vi "Binary to KLB(64-bit).vi"() -> ()   [LabVIEW 2013]
uses:
  File IO/KLB/VIs/Type Defs/KLB Settings Cluster.ctl
  File IO/KLB/VIs/Type Defs/KLB # of CPUs enum.ctl
  File IO/KLB/VIs/Type Defs/KLB compression type enum.ctl
  <vilib>/vision/Image Controls.llb/IMAQ Image.ctl
  File IO/KLB/KLB.lvlib
panel:
  in  "KLB Settings":T1={"Logical Cores"=enum."8", "pixelSize (um)"=[1.0, 1.0, 1.0, 1.0, 1.0], "blockSize"=[200, 197, 1, 1, 1], "compressionType"=enum."BZip2", "metadata"=""} {"pixelSize (um)" min=0.01 max=10 step=0.01 format="%.2f"}
  in  "Images per Chunk":u32=1
  out "Image":T4(plugin-control)
  out "KLB Conversion Time (ms)":u32=53091
  out "Image/Sector Size(bytes)":i64=3384359664
  in  "stop":bool
  out "Progress":u64(slide)=3579 max=5098 scale=0.0..3579.0
  out "Partial images in file?":bool
  out "# of Images":u32=3579
  out "error IO":errorcluster
  out "Height":u32=788
  out "Width":u32=1200
  in  "Created Image Path":path=path "G:/StreamingVideo/20150427_testStreamingVideoToDisk/09-25-2015_16-04-04-04 conv.klb"
  in  "Binary File":path=path "G:/StreamingVideo/20150427_testStreamingVideoToDisk/09-25-2015_16-04-04-04.bin"
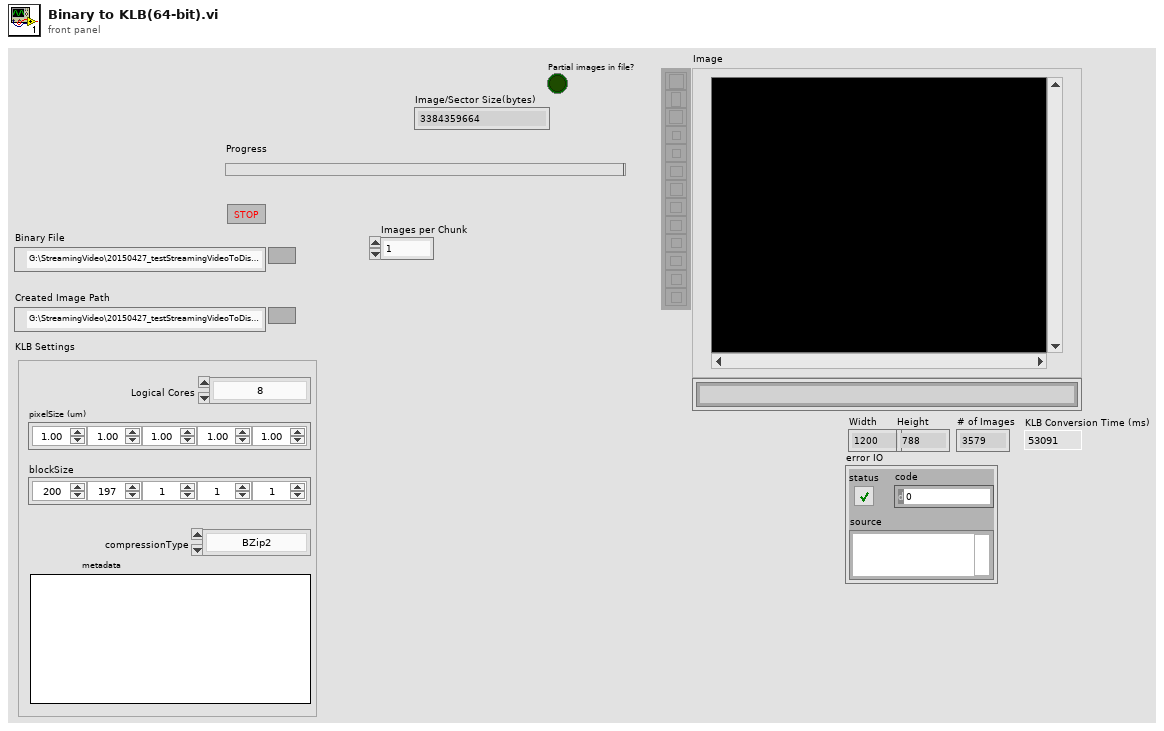
[diagram p1: front panel]
types:
  T1 = typedef "KLB.lvlib/KLB Settings Cluster.ctl" = cluster{"Logical Cores":T2, "pixelSize (um)":sgl[], "blockSize":u32[], "compressionType":T3, "metadata":string}
  T2 = typedef "KLB.lvlib/KLB # of CPUs enum.ctl" = enum16{"CPU 25%", "CPU 50%", "CPU 75%", "CPU All but 1", "1", "4", "8", "16"}
  T3 = typedef "KLB.lvlib/KLB compression type enum.ctl" = enum8{"Uncompressed", "BZip2"}
  T4 = typedef "IMAQ Image.ctl" = refnum<image>
  T5 = typedef "Mask ROI Cluster.ctl" = cluster{"left annulus":T6, "right annulus":T6, "Threshold Range":cluster{"Lower value":dbl, "Upper value":dbl}, "[Avg BG]":u8[], "Number of Sectors":u8, "Left ROI":T7, "Right ROI":T7, "Left Start Angle Duty Cycle":fxp<+,8,0>, "Left End Angle Duty Cycle":fxp<+,8,0>, "Right End Angle Duty Cycle":fxp<+,8,0>, "Right Start Angle Duty Cycle":fxp<+,8,0>, "[Sector ROIs]":T7[], "Consecutive Sector Threshold":u8}
  T6 = typedef "IMAQ Circle" = cluster{"Center X":i32, "Center Y":i32, "Inner Radius":i32, "Outer Radius":i32, "Start Angle":dbl, "End Angle":dbl}
  T7 = typedef "ROI Descriptor" = cluster{"Global Rectangle":i32[], "Contours":cluster{"ID":enum32{"External", "Internal"}, "Type":u32, "Coordinates":i32[]}[]}
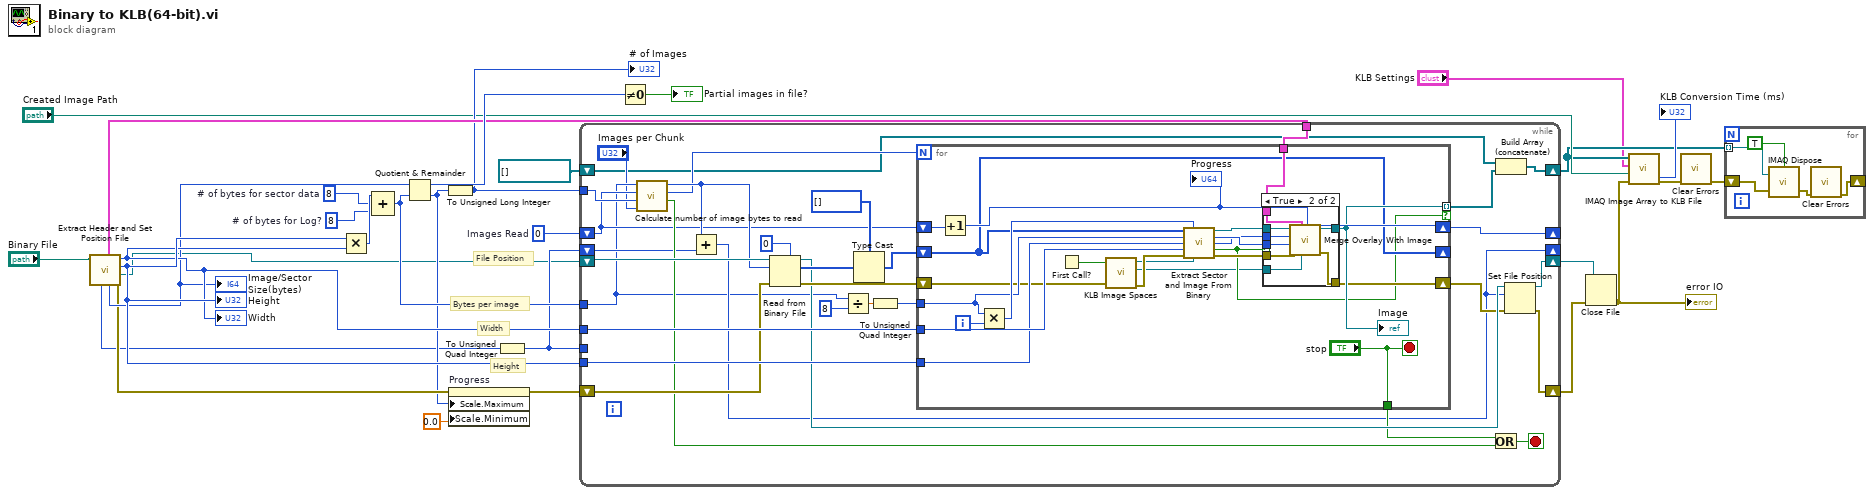
[diagram p0: block diagram]
diagram:
  w3 = u32 8  # # of bytes for Log?
  w16 = u32 0  # Images Read
  w22 = u32 8  # # of bytes for sector data
  # "Height"
  # "Width"
  # "Bytes per image"
  # "File Position"
  n1 = call "Extract Header and Set Position File.vi"("Binary File"="Binary File") -> ("error out"=w17:errorcluster, "refnum out"=w11:refnum<file>, "Height"=w20:u32, "Width"=w19:u32, "Image/Sector Size(bytes)"=w18:i64, "Mask ROI Out"=w12:T5, "Header Size"=w14:i32)  [unwired: 4 in]
  "Width" <- w19
  "Height" <- w20
  "Image/Sector Size(bytes)" <- w18
  n2 = Multiply(x=w20, y=w19) -> (x*y=w23:u32)
  n3 = Compound Arithmetic op=ADD(w23, w22, w3) -> (w21:u32)
  n4 = Quotient & Remainder(x=w18, y=w21) -> (x-y*floor(x/y)=w28:i64, floor(x/y)=w15:i64)
  n5 = To Unsigned Long Integer(number=w15) -> (unsigned 32bit integer=w10:u32)
  "# of Images" <- w10
  n6 = property on="Progress" class="Slide (strict)"(error in=w17, "Scale.Maximum"=w15, "Scale.Minimum"=0.0 ("Data Entry Limits:Minimum")) -> (error out=w26:errorcluster)  [unwired: 1 in, 1 out]
  n7 = To Unsigned Quad Integer(1:w14) -> (0:w13:u64)
  n8 = while {
    tunnel: w19 -> [w62]
    tunnel: w20 -> [w61]
    shift-right: [w54] -> w29
    shift-left: w26 -> [w59]
    shift-right: [w52] -> w27
    shift-left: w11 -> [w60]
    tunnel: w21 -> [w38]
    tunnel: w13 -> [_]
    shift-right: [w43] -> _
    shift-left: w16 -> [w44]
    tunnel: w10 -> [w51]
    shift-right: [w40] -> _
    shift-left: w13 -> [w48]
    tunnel: w12 -> [w39]
    shift-right: [w32] -> w6
    shift-left: T4[] [] -> [w31]
    stop <- w49 stop-if-true
    n9 = call "Calculate number of image bytes to read.vi"("Images per Chunk"="Images per Chunk", "# of total images"=w51, "Total Images Read"=w44, "# of bytes per image"=w38) -> ("All Images Read?"=w50:bool, "# of Images Read"=w45:u32, "# of bytes to read"=w47:u64)  [unwired: 5 in]
    n10 = Add(x=w47, y=w48) -> (x+y=w40:u64)
    n11 = Read from Binary File(5:u8 0, 8:w59, 10:w47, 11:w60) -> (0:w58:errorcluster, 2:w56:u8[], 3:w53:refnum<file>)  [unwired: 2 in, 1 out]
    n12 = Divide(x=w38, y=u32 8) -> (x/y=w36:dbl)
    n13 = Type Cast(type=u64[] [], x=w56) -> (*(type *) &x=w46:u64[])
    n14 = To Unsigned Quad Integer(1:w36) -> (0:w35:u64)
    n15 = for {
      N: w45 -> [_]
      tunnel: w62 -> [w82]
      tunnel: w61 -> [w81]
      shift-right: [w74] -> w43
      shift-left: w44 -> [w80]
      shift-right: [w71] -> w42
      shift-left: w58 -> [w67]
      tunnel: ["stop"] -> w41
      tunnel: w39 -> [w77]
      tunnel: w35 -> [w73]
      tunnel: [w72] -> w34 mode=indexing if=w68
      shift-right: [w69] -> _
      shift-left: w46 -> [w69]
      i -> [w84]
      stop <- "stop" stop-if-true
      n16 = Increment(x=w80) -> (x+1=w74:u32)
      "Progress" <- w74
      n17 = Multiply(x=w73, y=w84) -> (x*y=w83:u64)
      n18 = First Call?() -> (First Call?: T/F=w66:bool)
      n19 = call "KLB Image Spaces.vi"("error in (no error)"=w67, "Reset?"=w66) -> ("error out"=w65:errorcluster, "RGB Image"=w63:T4, "U8 Image"=w64:T4)  [unwired: 7 in]
      n20 = call "Extract Sector and Image From Binary.vi"("Binary Data(u64)"=w69, "Start Index"=w83, "# of u64 per image"=w73, "Height"=w81, "Width"=w82, "error in (no error)"=w65, "Image Destination"=w64) -> ("Image Out"=w78:T4, "Left Sector"=w76:u16, "Right Sector"=w75:u16, "Log?"=w68:bool, "error out"=w70:errorcluster)  [unwired: 4 in]
      n21 = case shown="True" w68 {
        tunnel: w78 -> [w86 w94]
        tunnel: w77 -> [_ w93]
        tunnel: w76 -> [_ w92]
        tunnel: w75 -> [_ w91]
        tunnel: [w86 w90] -> w72
        tunnel: [w85 w89] -> w71
        tunnel: w70 -> [w85 w88]
        tunnel: w63 -> [_ w87]
        frame False {
        }
        frame True {
          n22 = call "Merge Overlay With Image.vi"("Image RGB"=w87, "ROI Cluster"=w93, "Error in"=w88, "Left Edge"=w92, "Right Edge"=w91, "Image In"=w94) -> ("error out"=w89:errorcluster, "Image Out"=w90:T4)  [unwired: 4 in]
        }
      }
      "Image" <- w72
    }
    n23 = Or(x=w41, y=w50) -> (x .or. y?=w49:bool)
    n24 = Build Array (concatenate)(w31, w34) -> (w32:T4[])
    n25 = Set File Position(offset (in bytes) (0)=w40, refnum=w53, error in=w42) -> (refnum out=w52:refnum<file>, error out=w54:errorcluster)  [unwired: 1 in]
  }
  n26 = Not Equal To 0?(x=w28) -> (x != 0?=→"Partial images in file?":bool)
  n27 = Close File(refnum=w27, error in=w29) -> (error out=w5:errorcluster)  [unwired: 1 out]
  "error IO" <- w5
  n28 = call "IMAQ Image Array to KLB File.vi"("error in (no error)"=w5, "path"="Created Image Path", "KLB Settings"="KLB Settings", "Images to Compress"=w6) -> ("error out"=w7:errorcluster, "elapsed (ms)"=→"KLB Conversion Time (ms)":u32)  [unwired: 6 in]
  n29 = call <vilib>:"Clear Errors.vi"("error in (no error)"=w7) -> ("error out"=w4:errorcluster)  [unwired: 6 in]
  n30 = for {
    tunnel: w6 -> [w99] mode=indexing
    shift-right: [w95] -> _
    shift-left: w4 -> [w97]
    n31 = call "IMAQ Dispose"("All Images? (No)"=TRUE, "Image"=w99, "error in (no error)"=w97) -> ("error out"=w96:errorcluster)  [unwired: 3 in]
    n32 = call <vilib>:"Clear Errors.vi"("error in (no error)"=w96) -> ("error out"=w95:errorcluster)  [unwired: 6 in]
  }
